vi "ReceivePassInFuturePointTactic.vi"(7 "first call":bool, 8 "error in (no error)":errorcluster, 9 "Game in":refnum<class "Game.lvclass">, 10 "Robot":refnum<class "Robot.lvclass">, 11 "ReceivePassInFuturePointTactic in":refnum<class "ReceivePassInFuturePointTactic.lvclass">) -> (0 "error out":errorcluster, 2 "Robot out":refnum<class "Robot.lvclass">, 3 "ReceivePassInFuturePointTactic out":refnum<class "ReceivePassInFuturePointTactic.lvclass">)   [LabVIEW 2023, in "ReceivePassInFuturePointTactic.lvclass"]
uses:
  ReceivePassInFuturePointTactic.lvclass
  Robot_class/tactics.ctl
  GoToSkill_class/GoToSkill.lvclass
  HaltSkill_class/HaltSkill.lvclass
  Robot_class/Robot.lvclass
  Skillbook_class/Skillbook.lvclass
  Game_class/Game.lvclass
  Utilities_class/Utilities.lvclass
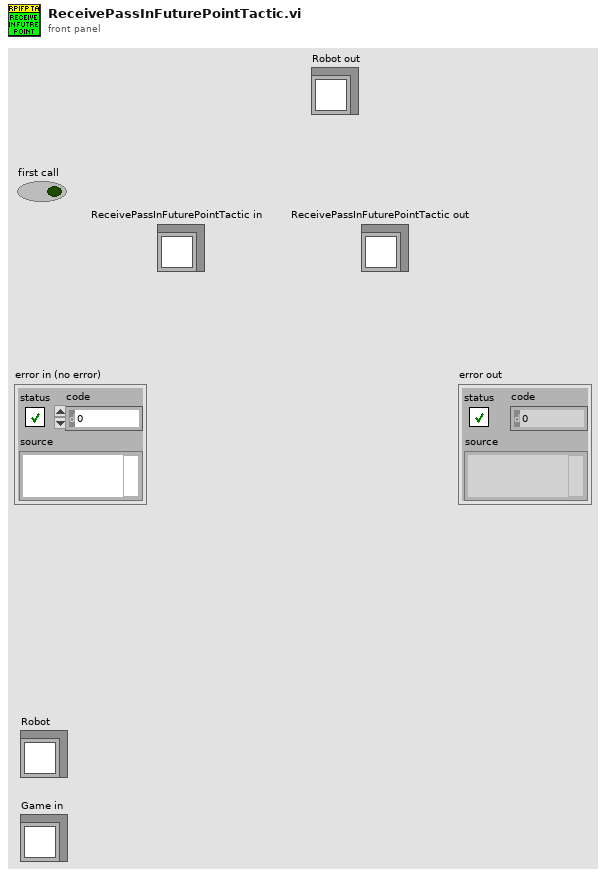
[diagram p1: front panel]
types:
  T1 = typedef "tactics.ctl" = enum16{"ReceivePassInFuturePoint", "Roller", "PrepareRollToPassRollerGoTo", "PrepareRollToPassReceiverGoTo", "WaitRoll", "PositionToRoll", "PenaltyAttacker", "PassObserver", "PenaltyDefense", "TableReceiverTactic", "Test", "DefendGoal", "Marker", "FollowAttacker", "DefendArea", "Shoot", "AttackerAimGoal", "AttackerBallOutOfField", "AttackerBlock", "AttackerStop", "Duelist", "Halt", "ZigZag", "GoTo", "Timeout", "KickToPassReceiver", "PositionToReceivePass", "DefendAreaVSS", "DefendGoalVSS", "KickVSS", "AttackVSS", "DispBallVSS", "PenaltyAttackVSS", "WaitPass"}
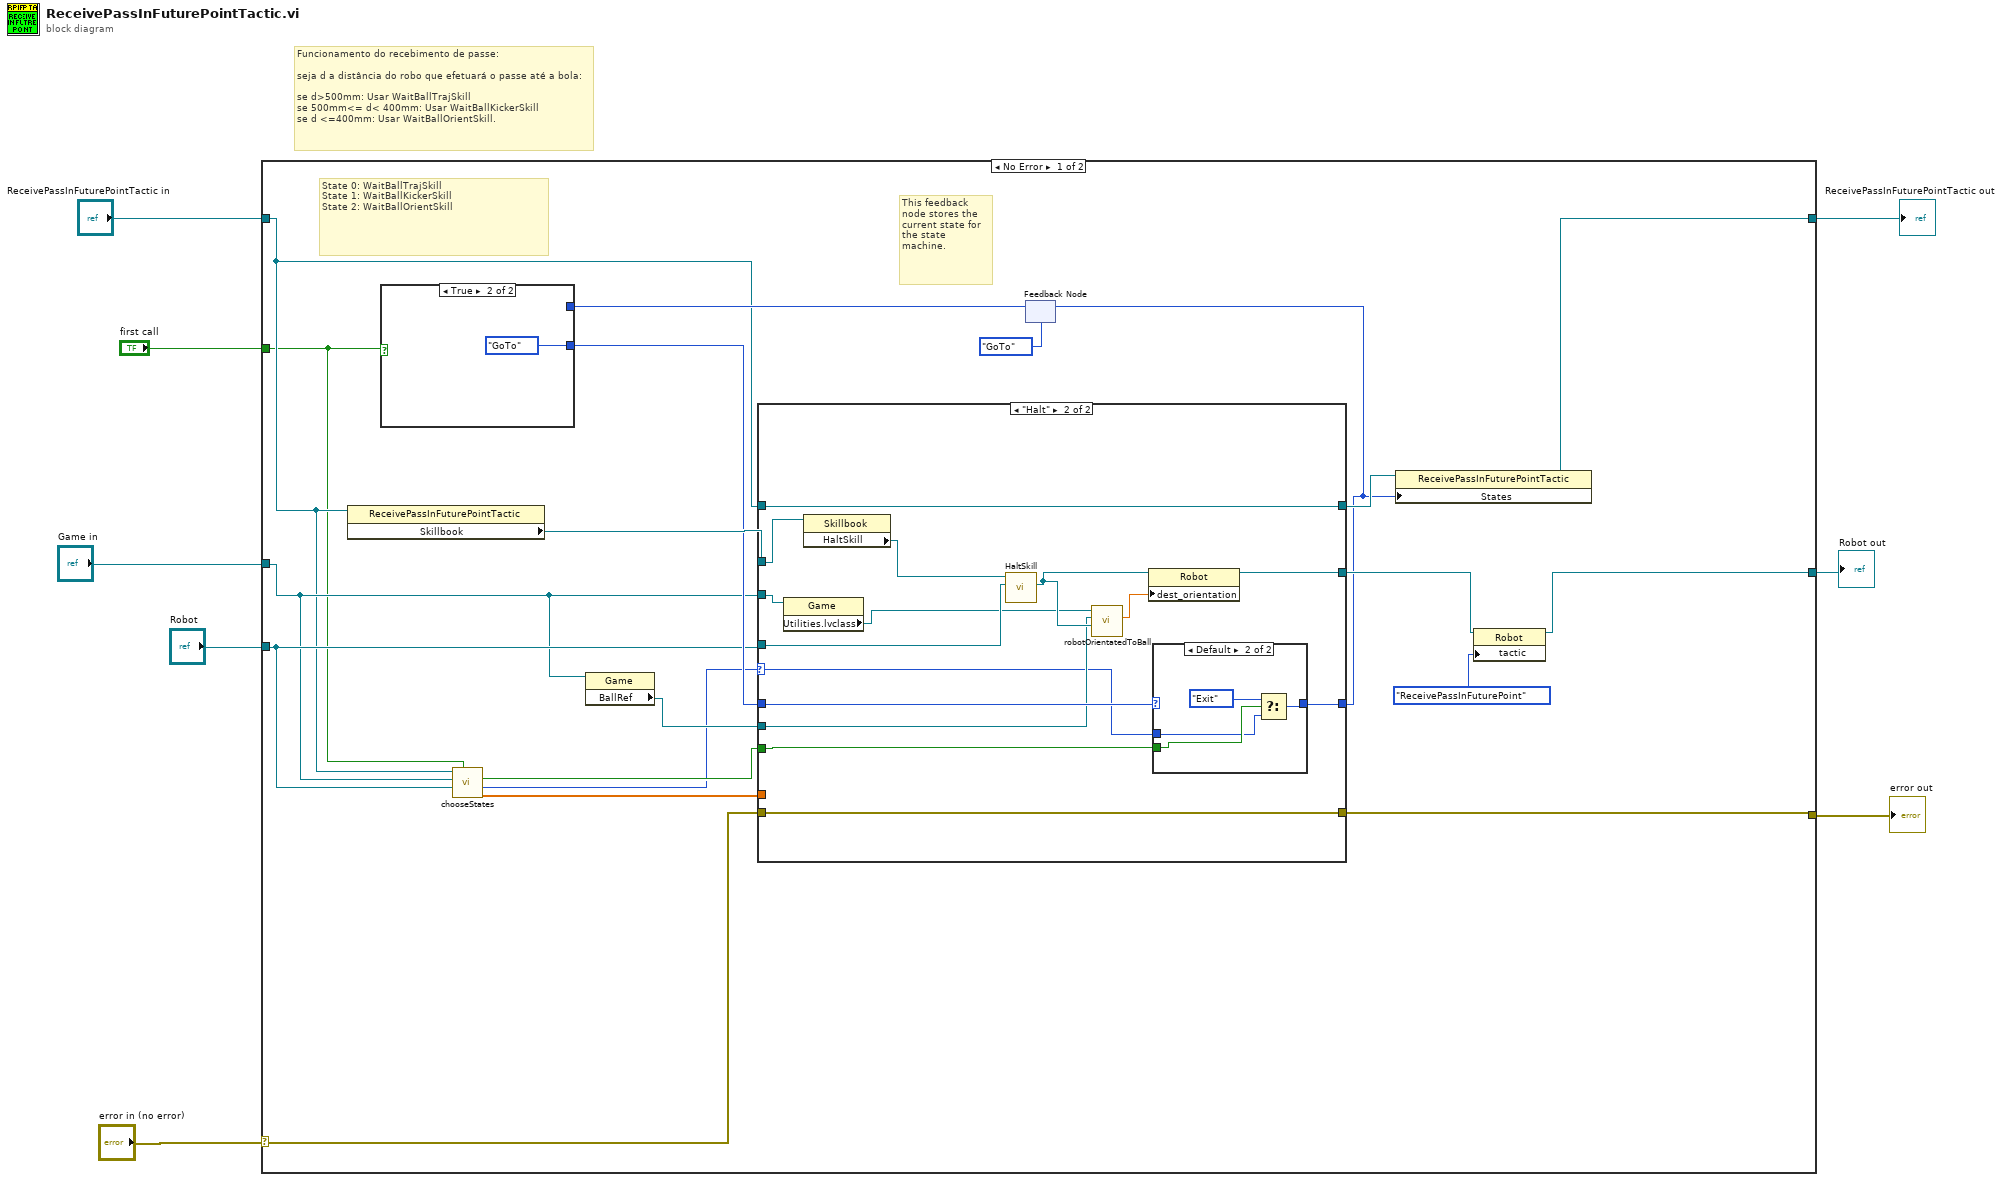
[diagram p0: block diagram]
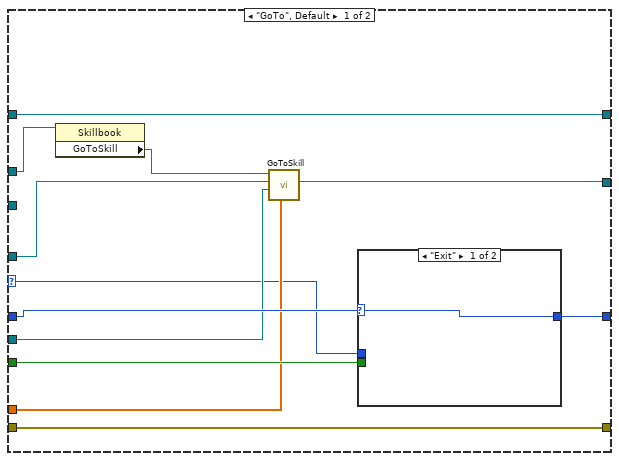
[diagram p3: hidden frame]
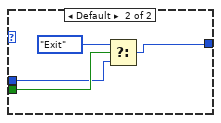
[diagram p4: hidden frame]
diagram:
  # "Funcionamento do recebimento de passe:\n\nseja d a distância do robo que efetuará o passe até a bola:\n\nse d>500mm: Usar WaitBallTrajSkill\nse 500mm<= d< 400mm: Usar WaitBallKickerSkill\nse d <=400mm: Usar WaitBallOrientSkill."
  n1 = case shown="No Error" "error in (no error)" {
    selector: "error in (no error)" -> [w24 w70]
    tunnel: [w23 w70] -> w7
    tunnel: [w21 w69] -> w1
    tunnel: "ReceivePassInFuturePointTactic in" -> [w12 w69]
    tunnel: "Game in" -> [w13 _]
    tunnel: "Robot" -> [w14 w68]
    tunnel: [w22 w68] -> w5
    tunnel: "first call" -> [w11 _]
    frame No Error {
      # "State 0: WaitBallTrajSkill\nState 1: WaitBallKickerSkill\nState 2: WaitBallOrientSkill"
      # "This feedback node stores the current state for the state machine."
      n2 = property class="ReceivePassInFuturePointTactic"(reference=w12) -> ("Skillbook"=w28:refnum<class "Skillbook.lvclass">)  [unwired: 1 in, 2 out]
      n3 = call "chooseStates.vi"("First call?"=w11, "Robot"=w14, "Game in"=w13, "ReceivePassInFuturePointTactic in"=w12) -> ("FuturePointToGo"=w9:dbl[], "StateToExecute"=w10:enum16{"Exit", "Halt", "GoTo"}, "ExitTactic?"=w18:bool)  [unwired: 4 in, 1 out]
      n4 = property class="Game"(reference=w13) -> ("BallRef"=w15:refnum<class "Ball.lvclass">)  [unwired: 1 in, 2 out]
      n5 = feedback #1(enum16{"Exit", "Halt", "GoTo"}."GoTo" ("States")) -> (w16:enum16{"Exit", "Halt", "GoTo"})
      n6 = case shown="True" w11 {
        tunnel: [w29 enum16{"Exit", "Halt", "GoTo"}."GoTo" ("States")] -> w17
        tunnel: w16 -> [w29 _]
        frame False {
        }
        frame True {
        }
      }
      n7 = case shown="\"Halt\"" w10 {
        selector: w10 -> [w31 w48]
        tunnel: w24 -> [w42 w62]
        tunnel: [w42 w62] -> w23
        tunnel: w28 -> [w41 w61]
        tunnel: w14 -> [w35 w59]
        tunnel: [w33 w55] -> w25
        tunnel: [w40 w56] -> w27
        tunnel: w12 -> [w40 w56]
        tunnel: w13 -> [_ w51]
        tunnel: [w38 w58] -> w19
        tunnel: w17 -> [w39 w57]
        tunnel: w15 -> [w36 w52]
        tunnel: w18 -> [w34 w49]
        tunnel: w9 -> [w32 _]
        frame "GoTo", Default {
          n8 = property class="Skillbook"(reference=w41) -> ("GoToSkill"=w37:refnum<class "GoToSkill.lvclass">)  [unwired: 1 in, 2 out]
          n9 = call "GoToSkill.vi"("Position"=w32, "BallRef"=w36, "Robot in"=w35, "GoToSkill in"=w37) -> ("Robot out"=w33:refnum<class "Robot.lvclass">)  [unwired: 5 in, 2 out]
          n10 = case shown="\"Exit\"" w39 {
            selector: w39 -> [w43 _]
            tunnel: [w43 w45] -> w38
            tunnel: w34 -> [_ w47]
            tunnel: w31 -> [_ w44]
            frame "Exit" {
            }
            frame Default {
              n11 = Select(t=enum16{"Exit", "Halt", "GoTo"}."Exit" ("States"), s=w47, f=w44) -> (s? t:f=w45:enum16{"Exit", "Halt", "GoTo"})
            }
          }
        }
        frame "Halt" {
          n12 = property class="Game"(reference=w51) -> ("Utilities.lvclass"=w50:refnum<class "Utilities.lvclass">)  [unwired: 1 in, 2 out]
          n13 = property class="Skillbook"(reference=w61) -> ("HaltSkill"=w60:refnum<class "HaltSkill.lvclass">)  [unwired: 1 in, 2 out]
          n14 = call-dynamic "HaltSkill.vi"("Robot"=w59, "HaltSkill in"=w60) -> ("Robot out"=w53:refnum<class "Robot.lvclass">)  [unwired: 7 in, 2 out]
          n15 = call "robotOrientatedToBall.vi"("Robot"=w53, "BallRef"=w52, "Utilities in"=w50) -> ("Orientation"=w54:dbl)  [unwired: 6 in, 2 out]
          n16 = property class="Robot"(reference=w53, "dest_orientation"=w54) -> (reference out=w55:refnum<class "Robot.lvclass">)  [unwired: 1 in, 1 out]
          n17 = case shown="Default" w57 {
            selector: w57 -> [w63 _]
            tunnel: [w63 w66] -> w58
            tunnel: w49 -> [_ w65]
            tunnel: w48 -> [_ w64]
            frame "Exit" {
            }
            frame Default {
              n18 = Select(t=enum16{"Exit", "Halt", "GoTo"}."Exit" ("States"), s=w65, f=w64) -> (s? t:f=w66:enum16{"Exit", "Halt", "GoTo"})
            }
          }
        }
      }
      n19 = feedback-in #1(w19) -> ()
      n20 = property class="ReceivePassInFuturePointTactic"(reference=w27, "States"=w19) -> (reference out=w21:refnum<class "ReceivePassInFuturePointTactic.lvclass">)  [unwired: 1 in, 1 out]
      n21 = property class="Robot"(reference=w25, "tactic"=tactics."ReceivePassInFuturePoint") -> (reference out=w22:refnum<class "Robot.lvclass">)  [unwired: 1 in, 1 out]
    }
    frame Error {
    }
  }
  "error out" <- w7
  "Robot out" <- w5
  "ReceivePassInFuturePointTactic out" <- w1
